vi "test_libssh2_userauth_keyboard_interactive_ex - no handler.vi"() -> ()   [LabVIEW 2017, in "integration_tests.lvlib"]
uses:
  integration_tests.lvlib
  libssh2/libssh2_session_handshake_tcp.vi
  libssh2/libssh2_init_default.vi
  <vilib>/Utility/tcp.llb/TCP Get Raw Net Object.vi
  libssh2/libssh2_session_handshake_socket.vi
  libssh2/libssh2.lvlib
  support/support.lvlib
  <vilib>/PNR/Transparent Assertions/Transparent Assertions/Transparent Assertions.lvlib
panel:
  out "error out":errorcluster
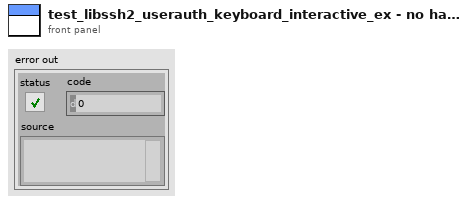
[diagram p1: front panel]
types:
  T1 = typedef "libssh2.lvlib/Session Refnum.ctl" = refnum<k1>
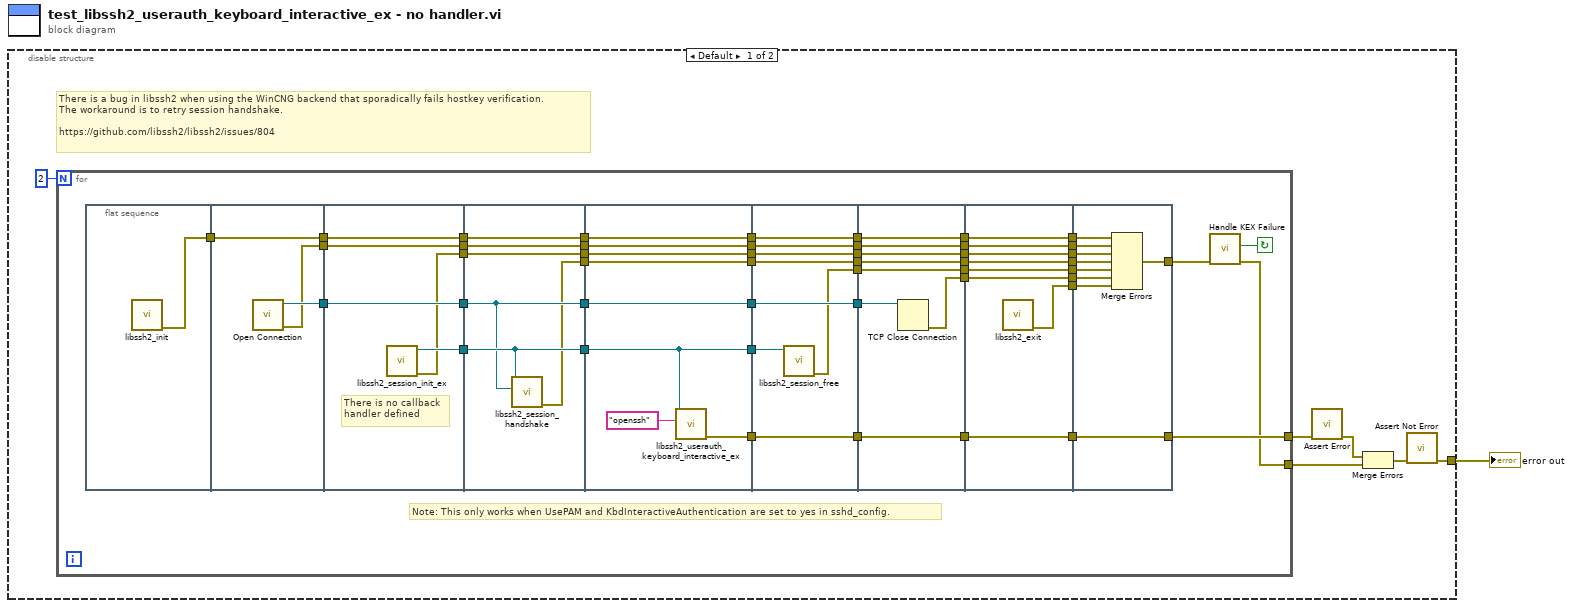
[diagram p0: block diagram]
diagram:
  n1 = disable-structure shown="Default" {
    disable-tunnel: [w7 _] -> w1
    frame condition #0 (active) {
      # "There is a bug in libssh2 when using the WinCNG backend that sporadically fails hostkey verification.\nThe workaround is to retry session handshake.\n\nhttps://github.com/libssh2/libssh2/issues/804"
      n2 = for {
        N: 2 -> [_]
        tunnel: [w11] -> w4
        tunnel: [w8] -> w6
        stop <- w9 continue-if-true
        # "Note: This only works when UsePAM and KbdInteractiveAuthentication are set to yes in sshd_config."
        n3 = flat-sequence {
          tunnel: [w56] -> w55
          tunnel: [w59] -> w54
          tunnel: w55 -> [w58]
          tunnel: [w58] -> w53
          tunnel: [w57] -> w52
          tunnel: w54 -> [w64]
          tunnel: [w64] -> w51
          tunnel: w53 -> [w63]
          tunnel: [w63] -> w50
          tunnel: w52 -> [w62]
          tunnel: [w62] -> w49
          tunnel: [w61] -> w48
          tunnel: [w60] -> w47
          tunnel: w51 -> [w66]
          tunnel: [w66] -> w46
          tunnel: w50 -> [w70]
          tunnel: [w70] -> w45
          tunnel: w49 -> [w69]
          tunnel: [w69] -> w44
          tunnel: [w68] -> w43
          tunnel: w48 -> [w68]
          tunnel: w47 -> [w67]
          tunnel: [w67] -> w42
          tunnel: [w65] -> w41
          tunnel: w46 -> [w78]
          tunnel: [w78] -> w40
          tunnel: w45 -> [w77]
          tunnel: [w77] -> w39
          tunnel: w44 -> [w76]
          tunnel: [w76] -> w38
          tunnel: w43 -> [w73]
          tunnel: w42 -> [w75]
          tunnel: [w75] -> w37
          tunnel: w41 -> [w74]
          tunnel: [w74] -> w36
          tunnel: [w73] -> w34
          tunnel: [w71] -> w35
          tunnel: w40 -> [w86]
          tunnel: [w86] -> w33
          tunnel: w39 -> [w85]
          tunnel: [w85] -> w32
          tunnel: w38 -> [w84]
          tunnel: [w84] -> w31
          tunnel: w37 -> [w83]
          tunnel: [w83] -> w30
          tunnel: w36 -> [w82]
          tunnel: [w82] -> w29
          tunnel: [w81] -> w28
          tunnel: [w80] -> w27
          tunnel: w35 -> [w80]
          tunnel: w34 -> [w79]
          tunnel: w33 -> [w94]
          tunnel: w32 -> [w93]
          tunnel: [w93] -> w26
          tunnel: w31 -> [w92]
          tunnel: [w92] -> w25
          tunnel: [w91] -> w24
          tunnel: w30 -> [w90]
          tunnel: [w90] -> w23
          tunnel: w29 -> [w89]
          tunnel: [w89] -> w22
          tunnel: [w88] -> w21
          tunnel: w28 -> [w88]
          tunnel: [w87] -> w20
          tunnel: w27 -> [w87]
          tunnel: w26 -> [w102]
          tunnel: [w102] -> w19
          tunnel: w25 -> [w101]
          tunnel: [w101] -> w18
          tunnel: w24 -> [w100]
          tunnel: [w100] -> w17
          tunnel: [w99] -> w16
          tunnel: w23 -> [w98]
          tunnel: [w98] -> w15
          tunnel: w22 -> [w97]
          tunnel: [w97] -> w14
          tunnel: [w96] -> w13
          tunnel: w21 -> [w96]
          tunnel: [w95] -> w12
          tunnel: w20 -> [w95]
          tunnel: w19 -> [w111]
          tunnel: w18 -> [w110]
          tunnel: w17 -> [w109]
          tunnel: w16 -> [w108]
          tunnel: w15 -> [w107]
          tunnel: w14 -> [w106]
          tunnel: w13 -> [w105]
          tunnel: w12 -> [w104]
          tunnel: [w104] -> w11
          tunnel: [w103] -> w10
          frame #0 {
            n4 = call-poly "libssh2_init.vi"() -> ("error out"=w56:errorcluster)  [unwired: 11 in]
          }
          frame #1 {
            n5 = call "Open Connection.vi"() -> ("error out"=w57:errorcluster, "connection ID"=w59:refnum<k5>)  [unwired: 10 in]
          }
          frame #2 {
            # "There is no callback\nhandler defined"
            n6 = call "libssh2_session_init_ex.vi"() -> ("error out"=w60:errorcluster, "session"=w61:T1)  [unwired: 10 in]
          }
          frame #3 {
            n7 = call-poly "libssh2_session_handshake.vi"("tcp connection"=w66, "session"=w68) -> ("error out"=w65:errorcluster)  [unwired: 9 in]
          }
          frame #4 {
            n8 = call "libssh2_userauth_keyboard_interactive_ex.vi"("username"="openssh", "session"=w73) -> ("error out"=w71:errorcluster)  [unwired: 9 in]
          }
          frame #5 {
            n9 = call "libssh2_session_free.vi"("session"=w79) -> ("error out"=w81:errorcluster)  [unwired: 10 in]
          }
          frame #6 {
            n10 = TCP Close Connection(connection ID=w94) -> (error out=w91:errorcluster)  [unwired: 2 in, 1 out]
          }
          frame #7 {
            n11 = call "libssh2_exit.vi"() -> ("error out"=w99:errorcluster)  [unwired: 11 in]
          }
          frame #8 {
            n12 = Merge Errors(w111, w110, w107, w106, w105, w109, w108) -> (w103:errorcluster)
          }
        }
        n13 = call "Handle KEX Failure.vi"("error in (no error)"=w10) -> ("error out"=w8:errorcluster, "KEX Failure"=w9:bool)  [unwired: 9 in]
      }
      n14 = call <vilib>:"Assert Error.vi"("error in (no error)"=w4) -> ("error out"=w2:errorcluster)  [unwired: 10 in]
      n15 = Merge Errors(w2, w6) -> (w3:errorcluster)
      n16 = call <vilib>:"Assert Not Error.vi"("error in (no error)"=w3) -> ("error out"=w7:errorcluster)  [unwired: 10 in]
    }
    frame condition #1 {
    }
  }
  "error out" <- w1
